vi "room align.vi"(8 "error in (no error)":errorcluster, 10 "Position in":T1, 11 "recycle":string) -> (0 "error out":errorcluster, 2 "side?":bool, 3 "Position out":T1)   [LabVIEW 2019]
uses:
  subVI/move/position cluster.ctl
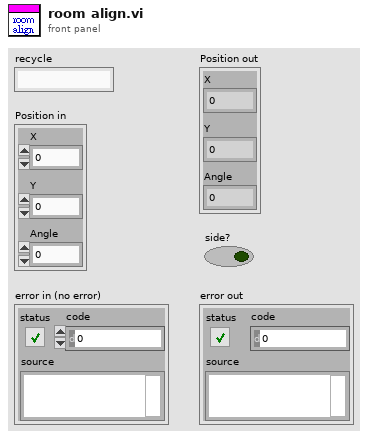
[diagram p1: front panel]
types:
  T1 = typedef "position cluster.ctl" = cluster{"X":dbl, "Y":dbl, "Angle":dbl}
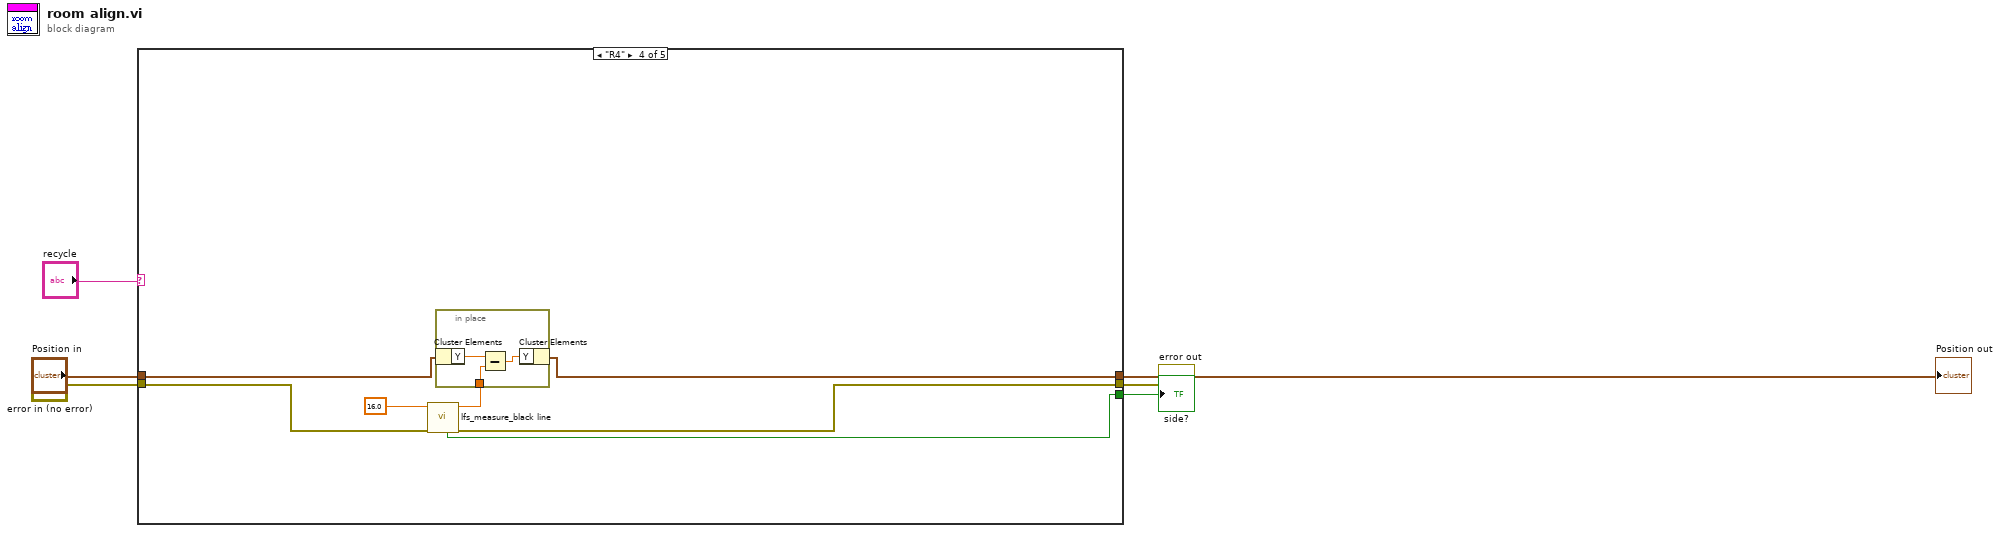
[diagram p0: block diagram]
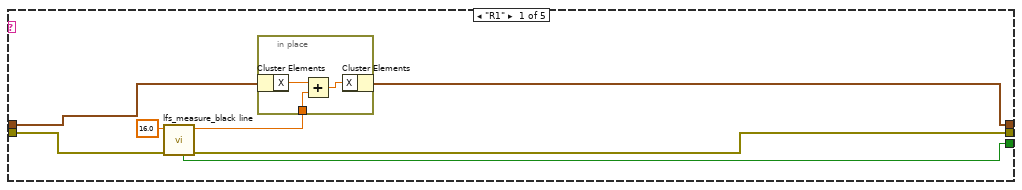
[diagram p2: hidden frame]
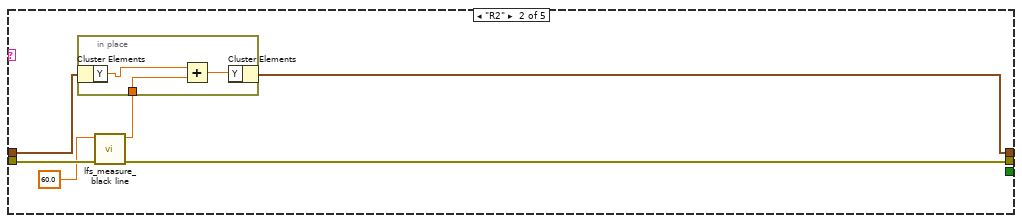
[diagram p3: hidden frame]
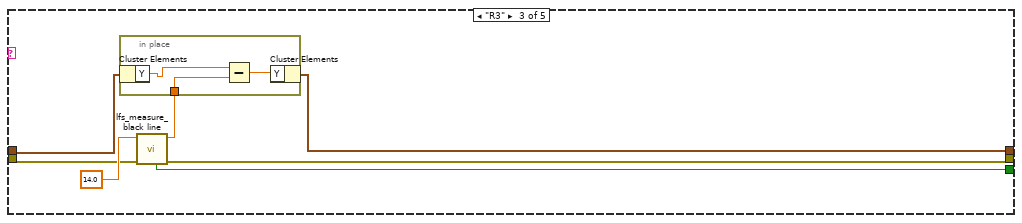
[diagram p4: hidden frame]
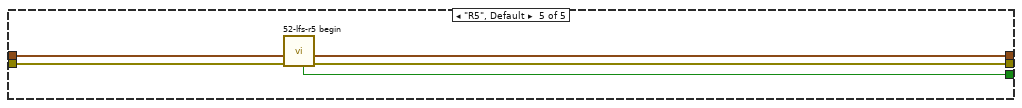
[diagram p5: hidden frame]
diagram:
  n1 = case shown="\"R4\"" "recycle" {
    tunnel: "error in (no error)" -> [w11 w22 w30 w38 w49]
    tunnel: "Position in" -> [w10 w20 w29 w39 w47]
    tunnel: [w9 w18 w28 w37 w50] -> w5
    tunnel: [w8 w17 w27 w40 w48] -> w4
    tunnel: [w7 _ w26 w36 w46] -> w6
    frame "R1" {
      n2 = call "lfs_measure_black line.vi"("error in (no error)"=w11, "limit"=16.0) -> ("error out"=w9:errorcluster, "move cm"=w13:dbl, "side?"=w7:bool)  [unwired: 6 in, 1 out]
      n3 = in-place {
        in-place-border: w13 -> [w15]
        n4 = in-place-cluster #1(w10) -> ("X"=w16:dbl)
        n5 = Add(x=w16, y=w15) -> (x+y=w14:dbl)
        n6 = in-place-cluster #1("X"=w14) -> (w8:T1)
      }
    }
    frame "R2" {
      n7 = call "lfs_measure_black line.vi"("error in (no error)"=w22, "limit"=60.0) -> ("error out"=w18:errorcluster, "move cm"=w19:dbl)  [unwired: 6 in, 2 out]
      n8 = in-place {
        in-place-border: w19 -> [w24]
        n9 = in-place-cluster #2(w20) -> ("Y"=w25:dbl)
        n10 = Add(x=w25, y=w24) -> (x+y=w23:dbl)
        n11 = in-place-cluster #2("Y"=w23) -> (w17:T1)
      }
    }
    frame "R3" {
      n12 = call "lfs_measure_black line.vi"("error in (no error)"=w30, "limit"=14.0) -> ("error out"=w28:errorcluster, "move cm"=w31:dbl, "side?"=w26:bool)  [unwired: 6 in, 1 out]
      n13 = in-place {
        in-place-border: w31 -> [w34]
        n14 = in-place-cluster #3(w29) -> ("Y"=w35:dbl)
        n15 = Subtract(x=w35, y=w34) -> (x-y=w33:dbl)
        n16 = in-place-cluster #3("Y"=w33) -> (w27:T1)
      }
    }
    frame "R4" {
      n17 = call "lfs_measure_black line.vi"("error in (no error)"=w38, "limit"=16.0) -> ("error out"=w37:errorcluster, "move cm"=w42:dbl, "side?"=w36:bool)  [unwired: 6 in, 1 out]
      n18 = in-place {
        in-place-border: w42 -> [w45]
        n19 = in-place-cluster #4(w39) -> ("Y"=w43:dbl)
        n20 = Subtract(x=w43, y=w45) -> (x-y=w44:dbl)
        n21 = in-place-cluster #4("Y"=w44) -> (w40:T1)
      }
    }
    frame "R5", Default {
      n22 = call "52-lfs-r5 begin.vi"("error in (no error)"=w49, "Position in"=w47) -> ("error out"=w50:errorcluster, "Position out"=w48:T1, "side?"=w46:bool)  [unwired: 7 in]
    }
  }
  "side?" <- w6
  "error out" <- w5
  "Position out" <- w4
